vi "Teleop Intake Control.vi"(1 "Manipulator Button Cluster":T2, 2 "Manipulator Axes":T1, 3 "Driver Axes":T1) -> ()   [LabVIEW 2015]
uses:
  Common Code/Gamepads/Button Cluster.ctl
  Common Code/Gamepads/Axes Cluster.ctl
  Common Code/Intake Commands.ctl
  Common Code/Change Detect Boolean.vi
  Robot Global Data.vi
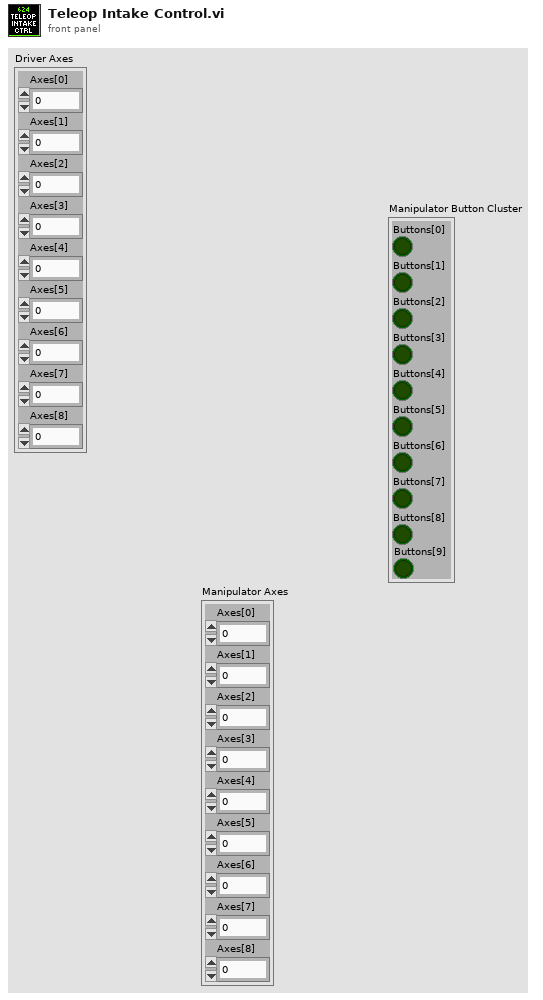
[diagram p1: front panel]
types:
  T1 = typedef "Axes Cluster.ctl" = cluster{"Axes[0]":dbl, "Axes[1]":dbl, "Axes[2]":dbl, "Axes[3]":dbl, "Axes[4]":dbl, "Axes[5]":dbl, "Axes[6]":dbl, "Axes[7]":dbl, "Axes[8]":dbl}
  T2 = typedef "Button Cluster.ctl" = cluster{"Buttons[0]":bool, "Buttons[1]":bool, "Buttons[2]":bool, "Buttons[3]":bool, "Buttons[4]":bool, "Buttons[5]":bool, "Buttons[6]":bool, "Buttons[7]":bool, "Buttons[8]":bool, "Buttons[9]":bool}
  T3 = typedef "Intake Commands.ctl" = enum16{"Zero", "Unload", "Load", "Drop low", "Idle"}
  T4 = enum16{"0", "1", "2", "3", "4", "5", "6", "7", "8", "9", "A", "B", "C", "D", "E", "F", "G", "H", "I", "J", "K", "L", "M", "N", "O", "P", "Q", "R", "S", "T", "U", "V", "W", "X", "Y", "Z", "F1", "F2", "F3", "F4", "F5", "F6", "F7", "F8", "F9", "F10", "F11", "F12", "F13", "F14", "F15", "ADD", "BACK", "BACKSLASH", "CAPITAL", "COMMA", "DECIMAL", "DELETE", "DIVIDE", "DOWN", "END", "EQUALS", "ESCAPE", "GRAVE (`)", "HOME", "INSERT", "LBRACKET", "LCONTROL", "LEFT", "L ALT", "LSHIFT", "LWIN", "MINUS", "MULTIPLY", "NEXT", "NUMLOCK", "NUMPAD_0", "NUMPAD_1", "NUMPAD_2", "NUMPAD_3", "NUMPAD_4", "NUMPAD_5", "NUMPAD_6", "NUMPAD_7", "NUMPAD_8", "NUMPAD_9", "PAUSE", "PERIOD", "PRIOR (PG UP)", "RBRACKET", "RCONTROL", "RETURN", "RIGHT", "R ALT", "RSHIFT", "RWIN", "SCROLL", "SEMICOLON", "SLASH", "SPACE", "SUBTRACT", "TAB", "UP", "ENTER (num pad)", "' (quote)"}
  T5 = typedef "Intake Mode.ctl" = enum16{"Manual", "Safe", "Auto"}
  T6 = typedef "Intake Commands Cluster.ctl" = cluster{"Intake Commands":T3, "Intake Mode":T5}
  T7 = typedef "Manual Intake Commands.ctl" = cluster{"Intake":bool, "Eject":bool, "Arm Angle":dbl, "Intake Override Speed":dbl, "Arm Override Speed":dbl, "Arm Speed":dbl, "Override Intake":bool, "Override Eject":bool, "Eject Override Speed":dbl, "Arm":bool, "Override Arm":bool, "Override Angle":bool}
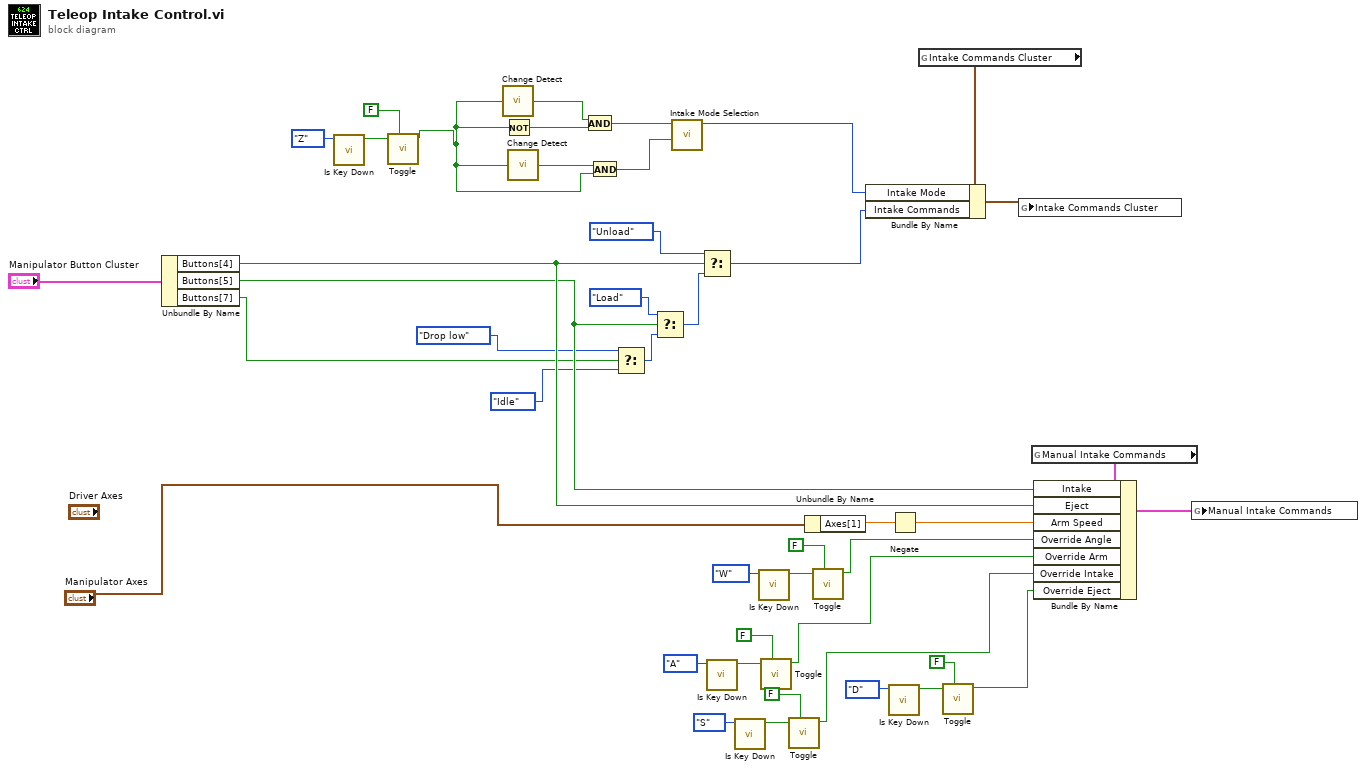
[diagram p0: block diagram]
diagram:
  n1 = Unbundle By Name("Manipulator Button Cluster") -> ("Buttons[4]"=w10:bool, "Buttons[5]"=w6:bool, "Buttons[7]"=w3:bool)
  n2 = call "Is Key Down.vi"("Key"=T4."Z") -> ("Key Down?"=w14:bool)  [unwired: 10 in]
  n3 = call "Toggle.vi"("Initial Value"=FALSE, "In"=w14) -> ("Toggled"=w11:bool)  [unwired: 9 in]
  n4 = call-poly "Change Detect.vi"("In"=w11) -> ("Changed?"=w20:bool)
  n5 = Not(x=w11) -> (.not. x?=w19:bool)
  n6 = call-poly "Change Detect.vi"("In"=w11) -> ("Changed?"=w18:bool)
  n7 = And(x=w20, y=w19) -> (x .and. y?=w16:bool)
  n8 = And(x=w18, y=w11) -> (x .and. y?=w15:bool)
  n9 = Select(t=Intake_Commands."Drop low" ("Intake Commands"), s=w3, f=Intake_Commands."Idle" ("Intake Commands")) -> (s? t:f=w4:T3)
  n10 = Select(t=Intake_Commands."Load" ("Intake Commands"), s=w6, f=w4) -> (s? t:f=w8:T3)
  n11 = call "Intake Mode Selection.vi"("Set To Manual?"=w15, "Set To Auto?"=w16) -> ("Mode"=w17:T5)  [unwired: 9 in]
  n12 = Select(t=Intake_Commands."Unload" ("Intake Commands"), s=w10, f=w8) -> (s? t:f=w7:T3)
  n13 = call "Is Key Down.vi"("Key"=T4."A") -> ("Key Down?"=w30:bool)  [unwired: 10 in]
  n14 = call "Is Key Down.vi"("Key"=T4."S") -> ("Key Down?"=w36:bool)  [unwired: 10 in]
  n15 = call "Is Key Down.vi"("Key"=T4."W") -> ("Key Down?"=w27:bool)  [unwired: 10 in]
  n16 = call "Toggle.vi"("Initial Value"=FALSE, "In"=w30) -> ("Toggled"=w23:bool)  [unwired: 9 in]
  n17 = call "Toggle.vi"("Initial Value"=FALSE, "In"=w36) -> ("Toggled"=w22:bool)  [unwired: 9 in]
  n18 = Unbundle By Name("Manipulator Axes") -> ("Axes[1]"=w40:dbl)
  n19 = call "Toggle.vi"("Initial Value"=FALSE, "In"=w27) -> ("Toggled"=w24:bool)  [unwired: 9 in]
  n20 = call "Is Key Down.vi"("Key"=T4."D") -> ("Key Down?"=w33:bool)  [unwired: 10 in]
  n21 = Negate(x=w40) -> (-x=w38:dbl)
  n22 = global read "Robot Global Data.vi" "Intake Commands Cluster"() -> (w43:T6)
  n23 = Bundle By Name(cluster=w43, "Intake Mode"=w17, "Intake Commands"=w7) -> (w42:T6)
  n24 = call "Toggle.vi"("Initial Value"=FALSE, "In"=w33) -> ("Toggled"=w21:bool)  [unwired: 9 in]
  n25 = global write "Robot Global Data.vi" "Intake Commands Cluster"(w42) -> ()
  n26 = global read "Robot Global Data.vi" "Manual Intake Commands"() -> (w37:T7)
  n27 = Bundle By Name(cluster=w37, "Intake"=w6, "Eject"=w10, "Arm Speed"=w38, "Override Angle"=w24, "Override Arm"=w23, "Override Intake"=w22, "Override Eject"=w21) -> (w39:T7)
  n28 = global write "Robot Global Data.vi" "Manual Intake Commands"(w39) -> ()
